vi "cake_size.vi"(7 "shape":enum16{"round", "rectangle", "triangle", ""}(ring), 8 "theta":dbl format="%#_13g", 9 "b":dbl format="%#_13g", 10 "a":dbl format="%#_13g", 11 "r":dbl format="%#_13g") -> (2 "size":dbl)   [LabVIEW 2023]
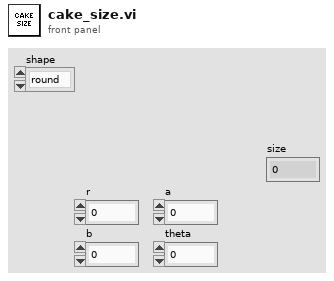
[diagram p1: front panel]
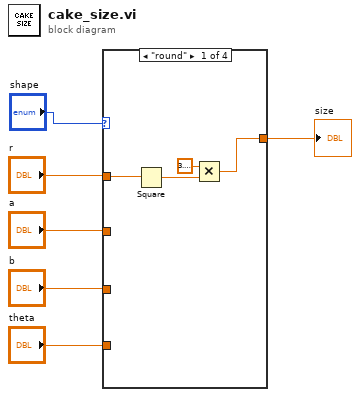
[diagram p0: block diagram]
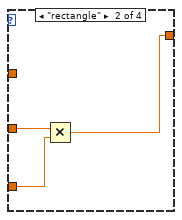
[diagram p2: hidden frame]
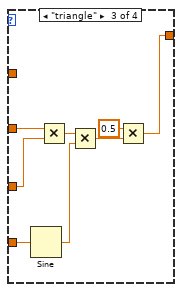
[diagram p3: hidden frame]
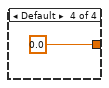
[diagram p4: hidden frame]
diagram:
  n1 = case shown="\"round\"" "shape" {
    tunnel: "r" -> [w8 _ _ _]
    tunnel: "a" -> [_ w13 w21 _]
    tunnel: "b" -> [_ w12 w20 _]
    tunnel: "theta" -> [_ _ w19 _]
    tunnel: [w7 w11 w14 0.0] -> w2
    frame "round" {
      n2 = Square(x=w8) -> (x^2=w9:dbl)
      n3 = Multiply(x=3.141592653589793, y=w9) -> (x*y=w7:dbl)
    }
    frame "rectangle" {
      n4 = Multiply(x=w13, y=w12) -> (x*y=w11:dbl)
    }
    frame "triangle" {
      n5 = Sine(x=w19) -> (sin(x)=w17:dbl)
      n6 = Multiply(x=w21, y=w20) -> (x*y=w18:dbl)
      n7 = Multiply(x=w18, y=w17) -> (x*y=w16:dbl)
      n8 = Multiply(x=0.5, y=w16) -> (x*y=w14:dbl)
    }
    frame Default {
    }
  }
  "size" <- w2
